vi "(Демо) Термометр.vi"(1 "Масштаб шкалы":bool) -> (0 "Температура":dbl(slide) scale=0.0..100.0)   [LabVIEW 2017]
doc: "This VI is the solution to an exercise in the LabVIEW Basics I course.\n\nIt measures temperature using the temperature sensor on the DAQ Signal Accessory."
panel:
  # "Град. C"
  # "Град. F"
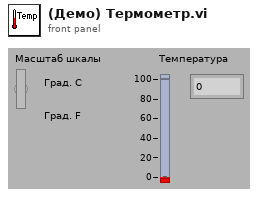
[diagram p1: front panel]
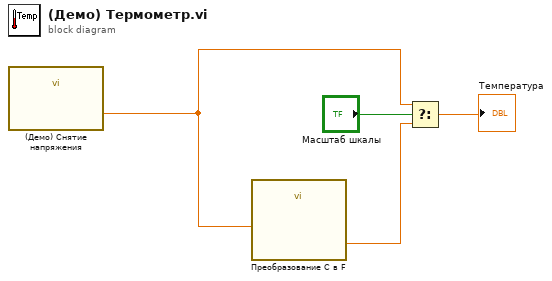
[diagram p0: block diagram]
diagram:
  n1 = call "(Демо) Снятие напряжения.vi"() -> ("Напряжение"=w1:dbl)  [unwired: 6 in, 1 out]
  n2 = call "Преобразование C в F.vi"("Град C"=w1) -> ("Град F"=w3:dbl)
  n3 = Select(t=w1, s="Масштаб шкалы", f=w3) -> (s? t:f=→"Температура":dbl)
